vi "BG_Subtraction.vi"(10 "Background Image":dbl[][](graph), 11 "Atom Image":dbl[][](graph)) -> (1 "Background Image Out":dbl[][](graph), 2 "Atom Image Out":dbl[][](graph), 3 "Atoms - BG":dbl[][](graph))   [LabVIEW 2013]
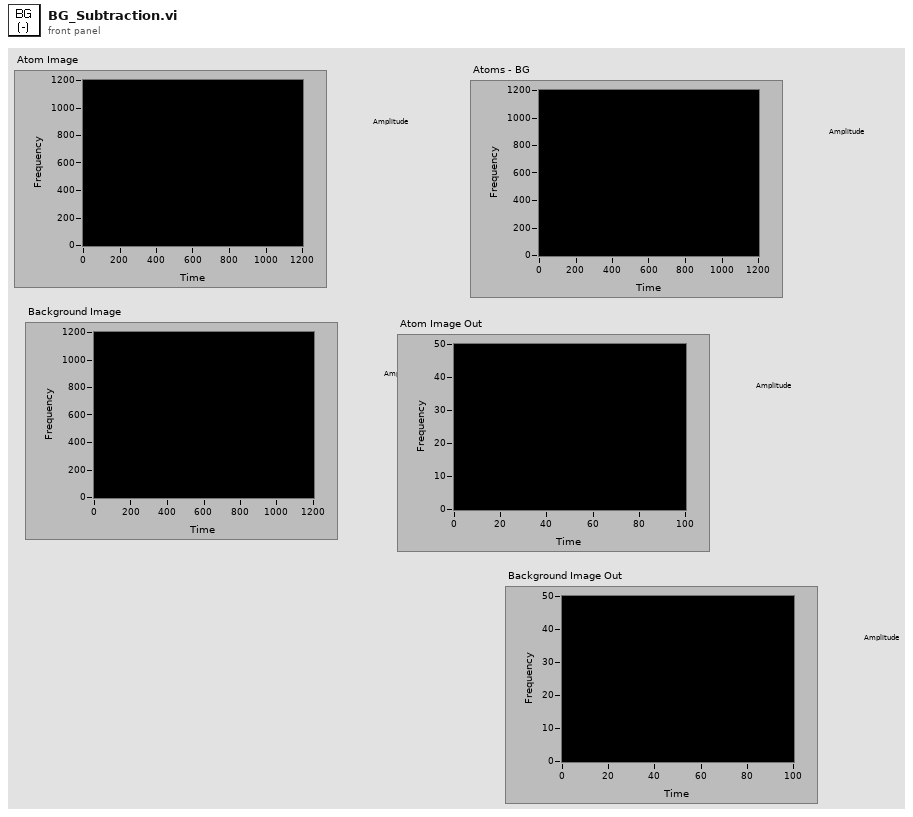
[diagram p1: front panel]
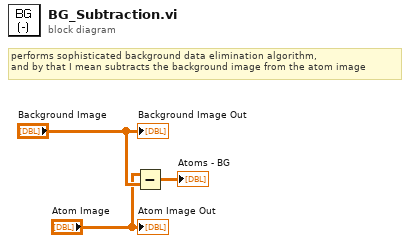
[diagram p0: block diagram]
diagram:
  # "performs sophisticated background data elimination algorithm,\nand by that I mean subtracts the background image from the atom image"
  n1 = Subtract(x="Atom Image", y="Background Image") -> (x-y=→"Atoms - BG":dbl[][])
  "Atom Image Out" <- "Atom Image"
  "Background Image Out" <- "Background Image"
